vi "报表.vi"() -> ()   [LabVIEW 2018]
uses:
  <vilib>/Utility/NIReport.llb/Report Type.ctl
  <vilib>/Utility/NIReport.llb/Append Report Text (str wrap).vi
  <vilib>/Utility/NIReport.llb/NI_report.lvclass
  <vilib>/Utility/NIReport.llb/NI_ReportGenerationCore.lvlib
panel:
  in  "按钮":bool
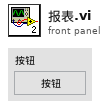
[diagram p1: front panel]
types:
  T1 = cluster{"position (Excel)":cluster{"row":i32, "column":i32}, "name (Excel)":string, "bookmark (Word)":string}
  T2 = typedef "NI_ReportGenerationCore.lvlib/Report Type.ctl" = enum16{"HTML", "Word", "Excel"}
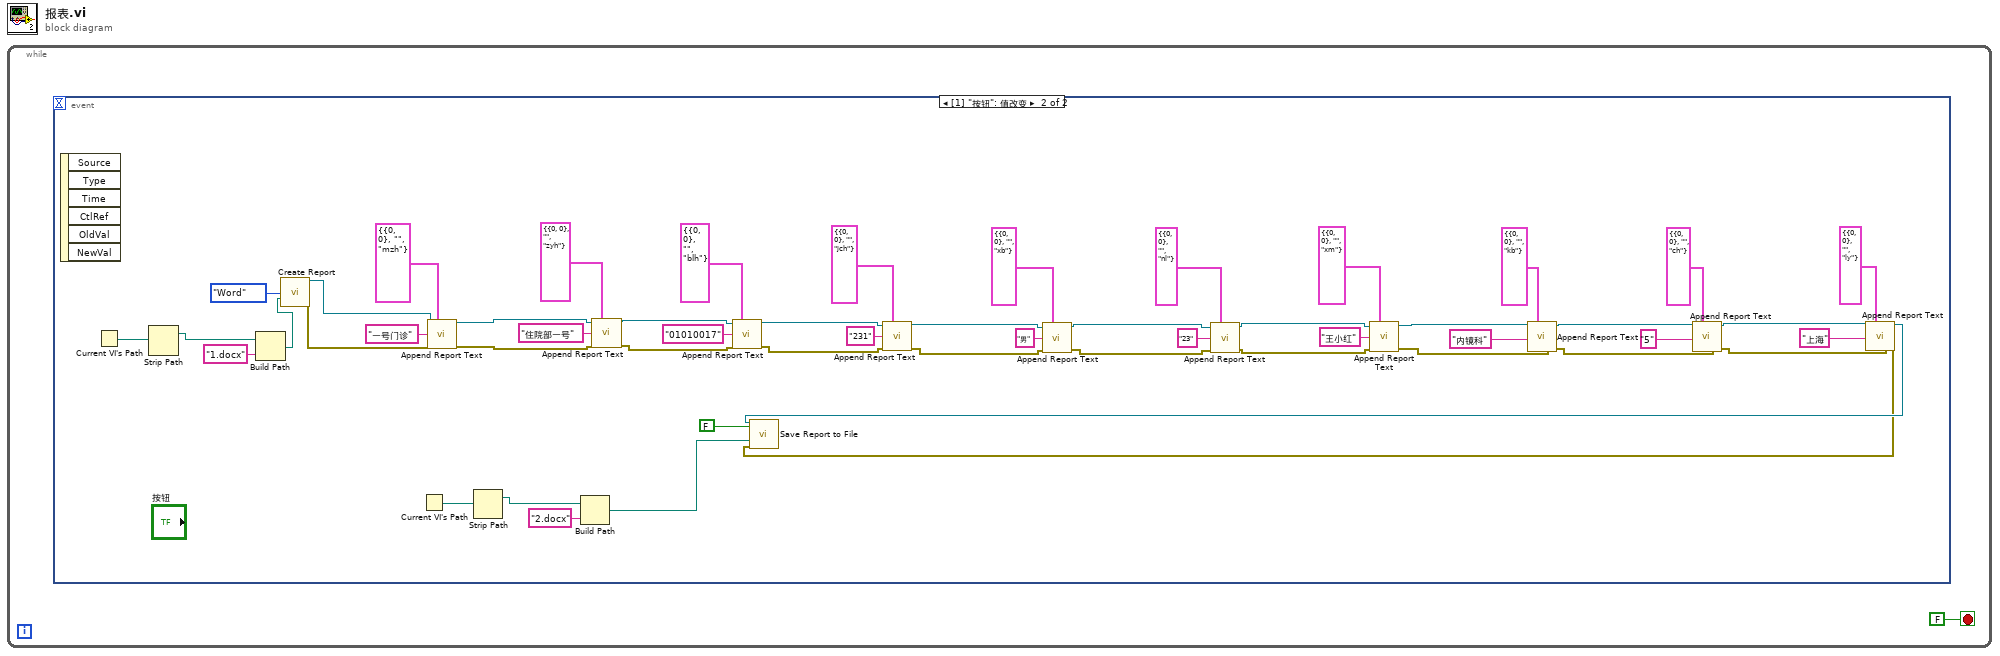
[diagram p0: block diagram]
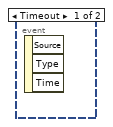
[diagram p2: hidden frame]
diagram:
  n1 = while {
    stop <- FALSE stop-if-true
    n2 = event shown="[1] \"按钮\": 值改变" {
      selector: _ -> [_ _]
      dyn-events: _ -> [_ _]
      timeout: _ -> [_ _]
      event Timeout {
        n3 = event-data() -> ()  [unwired: 1 in, 3 out]
      }
      event "按钮": Value Change {
        n4 = event-data() -> ()  [unwired: 1 in, 6 out]
        n5 = Current VI's Path() -> (path=w50:path)
        n6 = Strip Path(path=w50) -> (stripped path=w49:path)  [unwired: 1 out]
        n7 = Build Path(base path=w49, name or relative path="1.docx" ("名称或相对路径")) -> (appended path=w53:path)
        n8 = call <vilib>:"Create Report.vi"("report type"=Report_Type."Word" ("Report Type"), "template (empty)"=w53) -> ("report out"=w52:refnum<class "NI_report.lvclass">, "error out"=w51:errorcluster)  [unwired: 12 in]
        n9 = Current VI's Path() -> (path=w48:path)
        n10 = call-poly <vilib>:"Append Report Text.vi"("report in"=w52, "MS Office parameters"=T1 {"position (Excel)"={"row"=0, "column"=0}, "name (Excel)"="", "bookmark (Word)"="mzh"}, "text"="一号门诊", "error in (no error)"=w51) -> ("report out"=w44:refnum<class "NI_report.lvclass">, "error out"=w45:errorcluster)  [unwired: 8 in, 2 out]
        n11 = Strip Path(path=w48) -> (stripped path=w47:path)  [unwired: 1 out]
        n12 = Build Path(base path=w47, name or relative path="2.docx" ("名称或相对路径")) -> (appended path=w46:path)
        n13 = call-poly <vilib>:"Append Report Text.vi"("report in"=w44, "MS Office parameters"=T1 {"position (Excel)"={"row"=0, "column"=0}, "name (Excel)"="", "bookmark (Word)"="zyh"}, "text"="住院部一号", "error in (no error)"=w45) -> ("report out"=w33:refnum<class "NI_report.lvclass">, "error out"=w32:errorcluster)  [unwired: 8 in, 2 out]
        n14 = call-poly <vilib>:"Append Report Text.vi"("report in"=w33, "MS Office parameters"=T1 {"position (Excel)"={"row"=0, "column"=0}, "name (Excel)"="", "bookmark (Word)"="blh"}, "text"="01010017", "error in (no error)"=w32) -> ("report out"=w29:refnum<class "NI_report.lvclass">, "error out"=w28:errorcluster)  [unwired: 8 in, 2 out]
        n15 = call-poly <vilib>:"Append Report Text.vi"("report in"=w29, "MS Office parameters"=T1 {"position (Excel)"={"row"=0, "column"=0}, "name (Excel)"="", "bookmark (Word)"="jch"}, "text"="231", "error in (no error)"=w28) -> ("report out"=w25:refnum<class "NI_report.lvclass">, "error out"=w24:errorcluster)  [unwired: 8 in, 2 out]
        n16 = call-poly <vilib>:"Append Report Text.vi"("report in"=w25, "MS Office parameters"=T1 {"position (Excel)"={"row"=0, "column"=0}, "name (Excel)"="", "bookmark (Word)"="xb"}, "text"="男", "error in (no error)"=w24) -> ("report out"=w21:refnum<class "NI_report.lvclass">, "error out"=w20:errorcluster)  [unwired: 8 in, 2 out]
        n17 = call-poly <vilib>:"Append Report Text.vi"("report in"=w21, "MS Office parameters"=T1 {"position (Excel)"={"row"=0, "column"=0}, "name (Excel)"="", "bookmark (Word)"="nl"}, "text"="23", "error in (no error)"=w20) -> ("report out"=w17:refnum<class "NI_report.lvclass">, "error out"=w16:errorcluster)  [unwired: 8 in, 2 out]
        n18 = call-poly <vilib>:"Append Report Text.vi"("report in"=w17, "MS Office parameters"=T1 {"position (Excel)"={"row"=0, "column"=0}, "name (Excel)"="", "bookmark (Word)"="xm"}, "text"="王小红", "error in (no error)"=w16) -> ("report out"=w13:refnum<class "NI_report.lvclass">, "error out"=w12:errorcluster)  [unwired: 8 in, 2 out]
        n19 = call-poly <vilib>:"Append Report Text.vi"("report in"=w13, "MS Office parameters"=T1 {"position (Excel)"={"row"=0, "column"=0}, "name (Excel)"="", "bookmark (Word)"="kb"}, "text"="内镜科", "error in (no error)"=w12) -> ("report out"=w9:refnum<class "NI_report.lvclass">, "error out"=w8:errorcluster)  [unwired: 8 in, 2 out]
        n20 = call-poly <vilib>:"Append Report Text.vi"("report in"=w9, "MS Office parameters"=T1 {"position (Excel)"={"row"=0, "column"=0}, "name (Excel)"="", "bookmark (Word)"="ch"}, "text"="5", "error in (no error)"=w8) -> ("report out"=w5:refnum<class "NI_report.lvclass">, "error out"=w4:errorcluster)  [unwired: 8 in, 2 out]
        n21 = call-poly <vilib>:"Append Report Text.vi"("report in"=w5, "MS Office parameters"=T1 {"position (Excel)"={"row"=0, "column"=0}, "name (Excel)"="", "bookmark (Word)"="ly"}, "text"="上海", "error in (no error)"=w4) -> ("report out"=w3:refnum<class "NI_report.lvclass">, "error out"=w2:errorcluster)  [unwired: 8 in, 2 out]
        n22 = call-dynamic "Save Report to File.vi"("report in"=w3, "report file path"=w46, "prompt to replace? (F)"=FALSE, "error in (no error)"=w2) -> ()  [unwired: 10 in, 2 out]
      }
    }
  }
